vi "SinCos2.vi"() -> (8 "SinCos2":refnum<class "SinCos2.lvclass">)   [LabVIEW 2017, in "SinCos2.lvclass"]
uses:
  SinCos2.lvclass
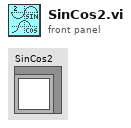
[diagram p1: front panel]
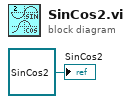
[diagram p0: block diagram]
diagram:
  "SinCos2" <- refnum<class "SinCos2.lvclass"> refnum ("SinCos2.lvclass")
